vi "FindMessageSet.vi"(7 "Actor":refnum<class "Actor.lvclass">) -> (3 "MessageSet":T1)   [LabVIEW 2020, in "jettl.lvlib" / "Base.lvlib" / "Actor.lvclass"]
uses:
  Actor.lvclass
  Message/Message.lvclass
  Actor.lvclass/Actor.ctl
  jettl.lvlib
  MessageSet.ctl
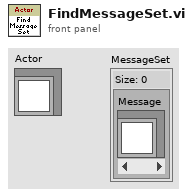
[diagram p1: front panel]
types:
  T1 = typedef "jettl.lvlib/MessageSet.ctl" = set{refnum<class "Message.lvclass">}
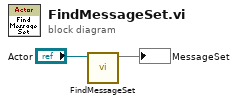
[diagram p0: block diagram]
diagram:
  n1 = call "FindMessageSet.vi"("ConcreteActor.lvclass"="Actor") -> ("MessageSet"=→"MessageSet":T1)  [unwired: 10 in]
